vi "CheckRowColumn.vi"(10 "RowColumn":i32[](array[numeric])) -> (1 "Complete":bool, 2 "Evaluation":i32)   [LabVIEW 2009, in "SudokuState.lvclass"]
uses:
  SudokuState.lvclass
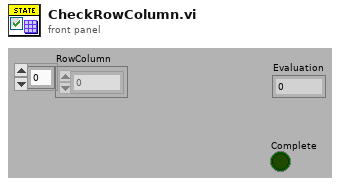
[diagram p1: front panel]
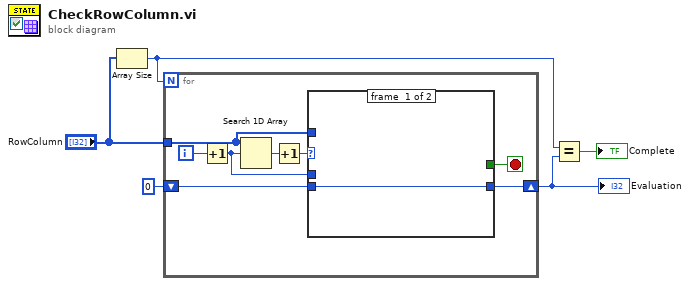
[diagram p0: block diagram]
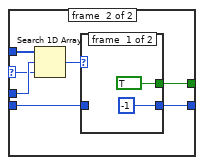
[diagram p2: hidden frame]
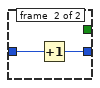
[diagram p3: hidden frame]
diagram:
  n1 = Array Size(array="RowColumn") -> (size(s)=w1:i32)
  n2 = for {
    N: w1 -> [_]
    tunnel: "RowColumn" -> [w12]
    shift-right: [w9] -> w3
    shift-left: 0 -> [w10]
    i -> [w13]
    stop <- w8 stop-if-true
    n3 = Increment(x=w13) -> (x+1=w11:i32)
    n4 = Search 1D Array(1D array=w12, element=w11) -> (index of element=w7:i32)  [unwired: 1 in]
    n5 = Increment(x=w7) -> (x+1=w6:i32)
    n6 = case shown="0" w6 {
      selector: w6 -> [_ w19]
      tunnel: w12 -> [_ w21]
      tunnel: w11 -> [_ w20]
      tunnel: w10 -> [w14 w17]
      tunnel: [w14 w16] -> w9
      tunnel: [_ w15] -> w8
      frame #0 {
      }
      frame #1 {
        n7 = Search 1D Array(1D array=w21, element=w20, start index (0)=w19) -> (index of element=w18:i32)
        n8 = case shown="-1" w18 {
          tunnel: w17 -> [_ w25]
          tunnel: [-1 w24] -> w16
          tunnel: [TRUE _] -> w15
          frame #0 {
          }
          frame #1 {
            n9 = Increment(x=w25) -> (x+1=w24:i32)
          }
        }
      }
    }
  }
  "Evaluation" <- w3
  n10 = Equal?(x=w1, y=w3) -> (x = y?=→"Complete":bool)
